vi "PRUEBA.vi"() -> ()   [LabVIEW 2022 SP3]
panel:
  out "ID String 3":string
  out "Data String 3":string
  in  "ID ESPERADO STRING 3":string
  in  "string 3":string
  in  "ID 3":string
  out "ID String 2":string
  out "Data String 2":string
  in  "ID ESPERADO STRING 2":string
  in  "string 2":string
  in  "ID 2":string
  out "ID String":string
  out "Data String":string
  in  "ID ESPERADO STRING":string
  in  "interface":refnum<k21>
  in  "string":string
  in  "ID":string
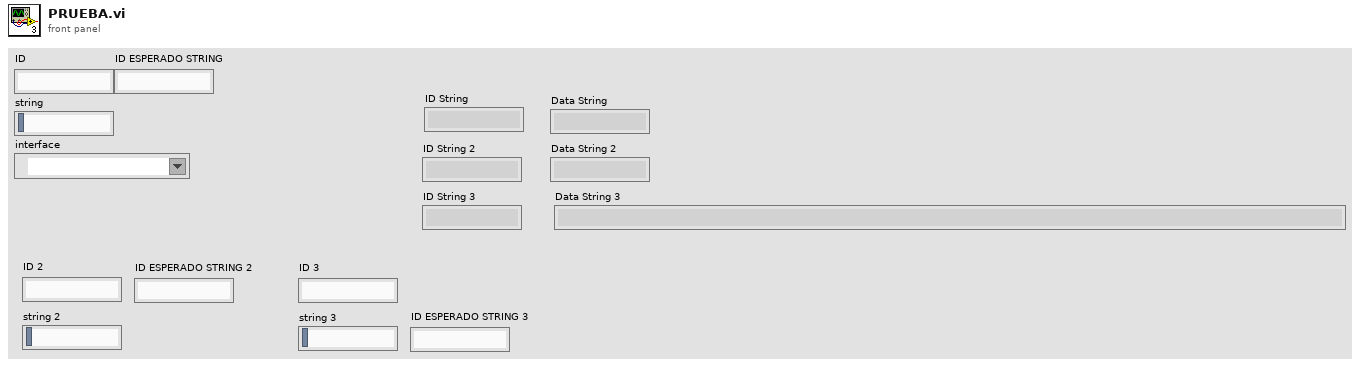
[diagram p1: front panel]
types:
  T1 = typedef "XNET Frame CAN.ctl" = cluster{"timestamp":timestamp, "payload":u8[], "identifier":u32, "type":T2, "extended?":bool, "echo?":bool}
  T2 = typedef "XNET Frame Type CAN.ctl" = u8
  T3 = cluster{"data[0]":T1, "data[1]":T1, "data[2]":T1, "data[3]":T1, "data[4]":T1, "data[5]":T1, "data[6]":T1, "data[7]":T1, "data[8]":T1}
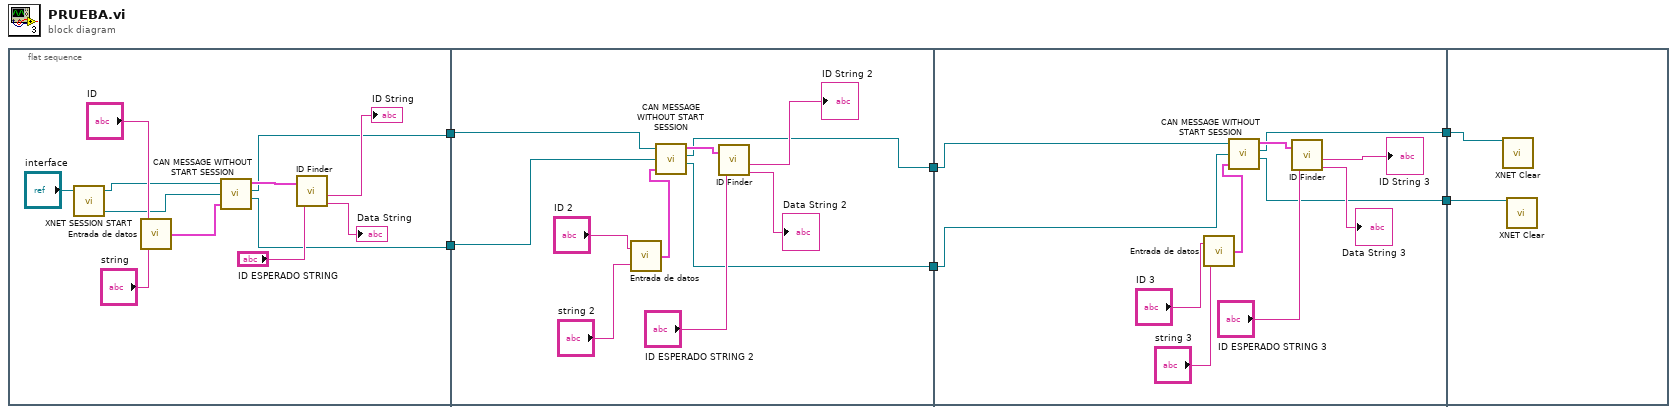
[diagram p0: block diagram]
diagram:
  n1 = flat-sequence {
    tunnel: [w8] -> w6
    tunnel: [w7] -> w5
    tunnel: [w22] -> w4
    tunnel: [w21] -> w3
    tunnel: w5 -> [w20]
    tunnel: w6 -> [w19]
    tunnel: w3 -> [w33]
    tunnel: w4 -> [w32]
    tunnel: [w31] -> w2
    tunnel: [w30] -> w1
    tunnel: w2 -> [w42]
    tunnel: w1 -> [w41]
    frame #0 {
      n2 = call "XNET SESSION START.vi"("interface"="interface") -> ("Read"=w9:refnum<k21>, "Write"=w10:refnum<k21>)  [unwired: 2 in, 1 out]
      n3 = call "Entrada de datos.vi"("string"="string", "ID"="ID") -> ("CAN frame"=w15:T1)
      n4 = call "CAN MESSAGE WITHOUT START SESSION.vi"("Write"=w10, "Read"=w9, "CAN frame"=w15) -> ("cluster"=w14:T3, "Write"=w7:refnum<k21>, "Read"=w8:refnum<k21>)  [unwired: 1 out]
      n5 = call "ID Finder.vi"("cluster"=w14, "ID ESPERADO STRING"="ID ESPERADO STRING") -> ("ID String"=→"ID String":string, "Data String"=→"Data String":string)  [unwired: 4 out]
    }
    frame #1 {
      n6 = call "Entrada de datos.vi"("string"="string 2", "ID"="ID 2") -> ("CAN frame"=w25:T1)
      n7 = call "CAN MESSAGE WITHOUT START SESSION.vi"("Write"=w20, "Read"=w19, "CAN frame"=w25) -> ("cluster"=w26:T3, "Write"=w22:refnum<k21>, "Read"=w21:refnum<k21>)  [unwired: 1 out]
      n8 = call "ID Finder.vi"("cluster"=w26, "ID ESPERADO STRING"="ID ESPERADO STRING 2") -> ("ID String"=→"ID String 2":string, "Data String"=→"Data String 2":string)  [unwired: 4 out]
    }
    frame #2 {
      n9 = call "Entrada de datos.vi"("string"="string 3", "ID"="ID 3") -> ("CAN frame"=w36:T1)
      n10 = call "CAN MESSAGE WITHOUT START SESSION.vi"("Write"=w32, "Read"=w33, "CAN frame"=w36) -> ("cluster"=w37:T3, "Write"=w31:refnum<k21>, "Read"=w30:refnum<k21>)  [unwired: 1 out]
      n11 = call "ID Finder.vi"("cluster"=w37, "ID ESPERADO STRING"="ID ESPERADO STRING 3") -> ("ID String"=→"ID String 3":string, "Data String"=→"Data String 3":string)  [unwired: 4 out]
    }
    frame #3 {
      n12 = call <vilib>:"XNET Clear.vi"("session in"=w42) -> ()  [unwired: 14 in, 1 out]
      n13 = call <vilib>:"XNET Clear.vi"("session in"=w41) -> ()  [unwired: 14 in, 1 out]
    }
  }
